vi "Dynamic Circle Find.vi"(8 "error in":errorcluster, 9 "Range":cluster{"Start":sgl, "Count":sgl}={"Start"=0.0, "Count"=255.0}, 10 "Treatment":T1, 11 "Images":T3) -> (0 "error out":errorcluster, 2 "Circle":T4, 3 "Found":bool)   [LabVIEW 2015]
uses:
  controls/Results.ctl
  controls/Images.ctl
  <vilib>/vision/Image Controls.llb/IMAQ Image.ctl
  controls/Treatment Parameters.ctl
  <vilib>/vision/NI_Vision_Development_Module.lvlib
panel:
  out "Array":sgl[][](array[numeric])
  out "Template":T2(plugin-control)
  out "Buffer":T2(plugin-control)
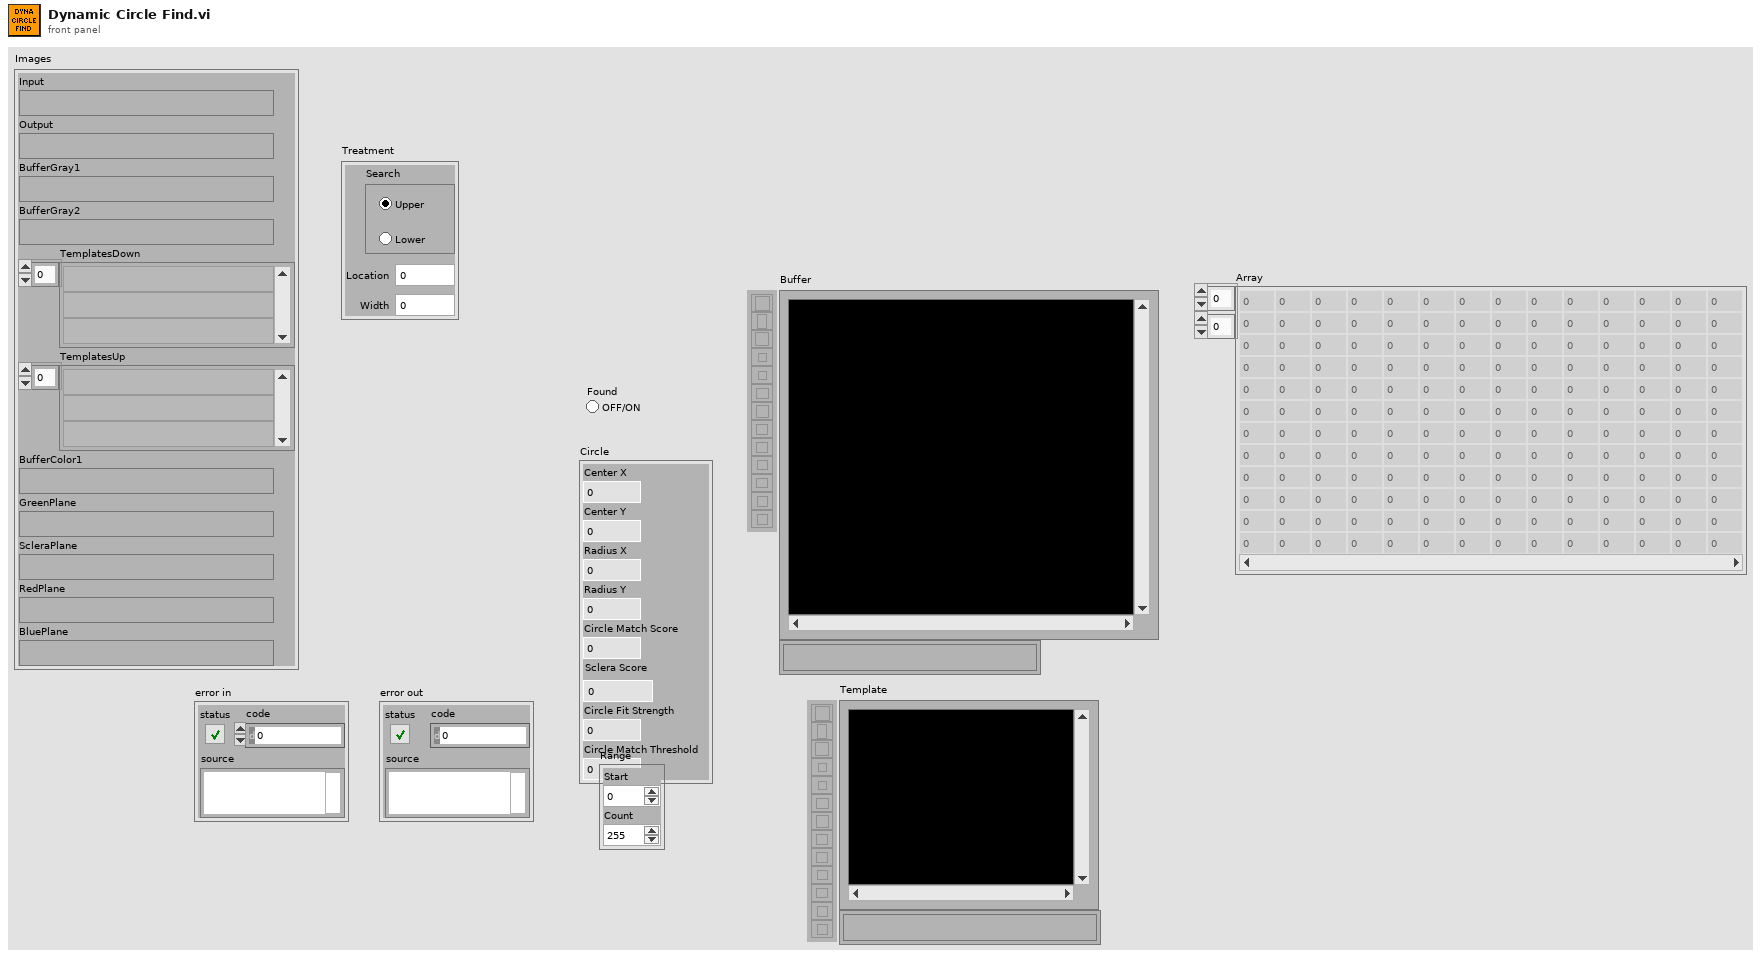
[diagram p1: front panel]
types:
  T1 = typedef "Treatment Parameters.ctl" = cluster{"Location":dbl, "Width":dbl, "Search":enum32{"Upper", "Lower"}}
  T2 = typedef "IMAQ Image.ctl" = refnum<image>
  T3 = typedef "Images.ctl" = cluster{"Input":T2, "Output":T2, "BufferGray1":T2, "BufferGray2":T2, "TemplatesDown":T2[], "TemplatesUp":T2[], "BufferColor1":T2, "GreenPlane":T2, "ScleraPlane":T2, "RedPlane":T2, "BluePlane":T2}
  T4 = typedef "Results.ctl" = cluster{"Center X":i32, "Center Y":i32, "Radius X":i32, "Radius Y":i32, "Circle Match Score":i32, "Sclera Score":dbl, "Circle Fit Strength":i32, "Circle Match Threshold":i32}
  T5 = cluster{"Global Rectangle":i32[], "Contours":cluster{"ID":enum32{"External", "Internal"}, "Type":u32, "Coordinates":i32[]}[]}
  T6 = cluster{"Number of Matches Requested":i32, "Minimum Match Score":sgl, "Angle Ranges":cluster{"Start Angle":sgl, "End Angle":sgl}[]}
  T7 = cluster{"histogram":u32[], "Minimal Value":sgl, "Maximal Value":sgl, "Starting Value":sgl, "Interval Width":sgl, "Mean Value":sgl, "Standard  Variation":sgl, "Area (pixels)":i32}
  T8 = typedef "Image Type" = u32
  T9 = cluster{"Position":cluster{"x":sgl, "y":sgl}, "Angle":sgl, "Scale":sgl, "Score":sgl, "Bounding Box":cluster{"x":sgl, "y":sgl}[]}[]
  T10 = cluster{"Position":cluster{"x":sgl, "y":sgl}, "Angle":sgl, "Scale":sgl, "Score":sgl, "Bounding Box":cluster{"x":sgl, "y":sgl}[]}
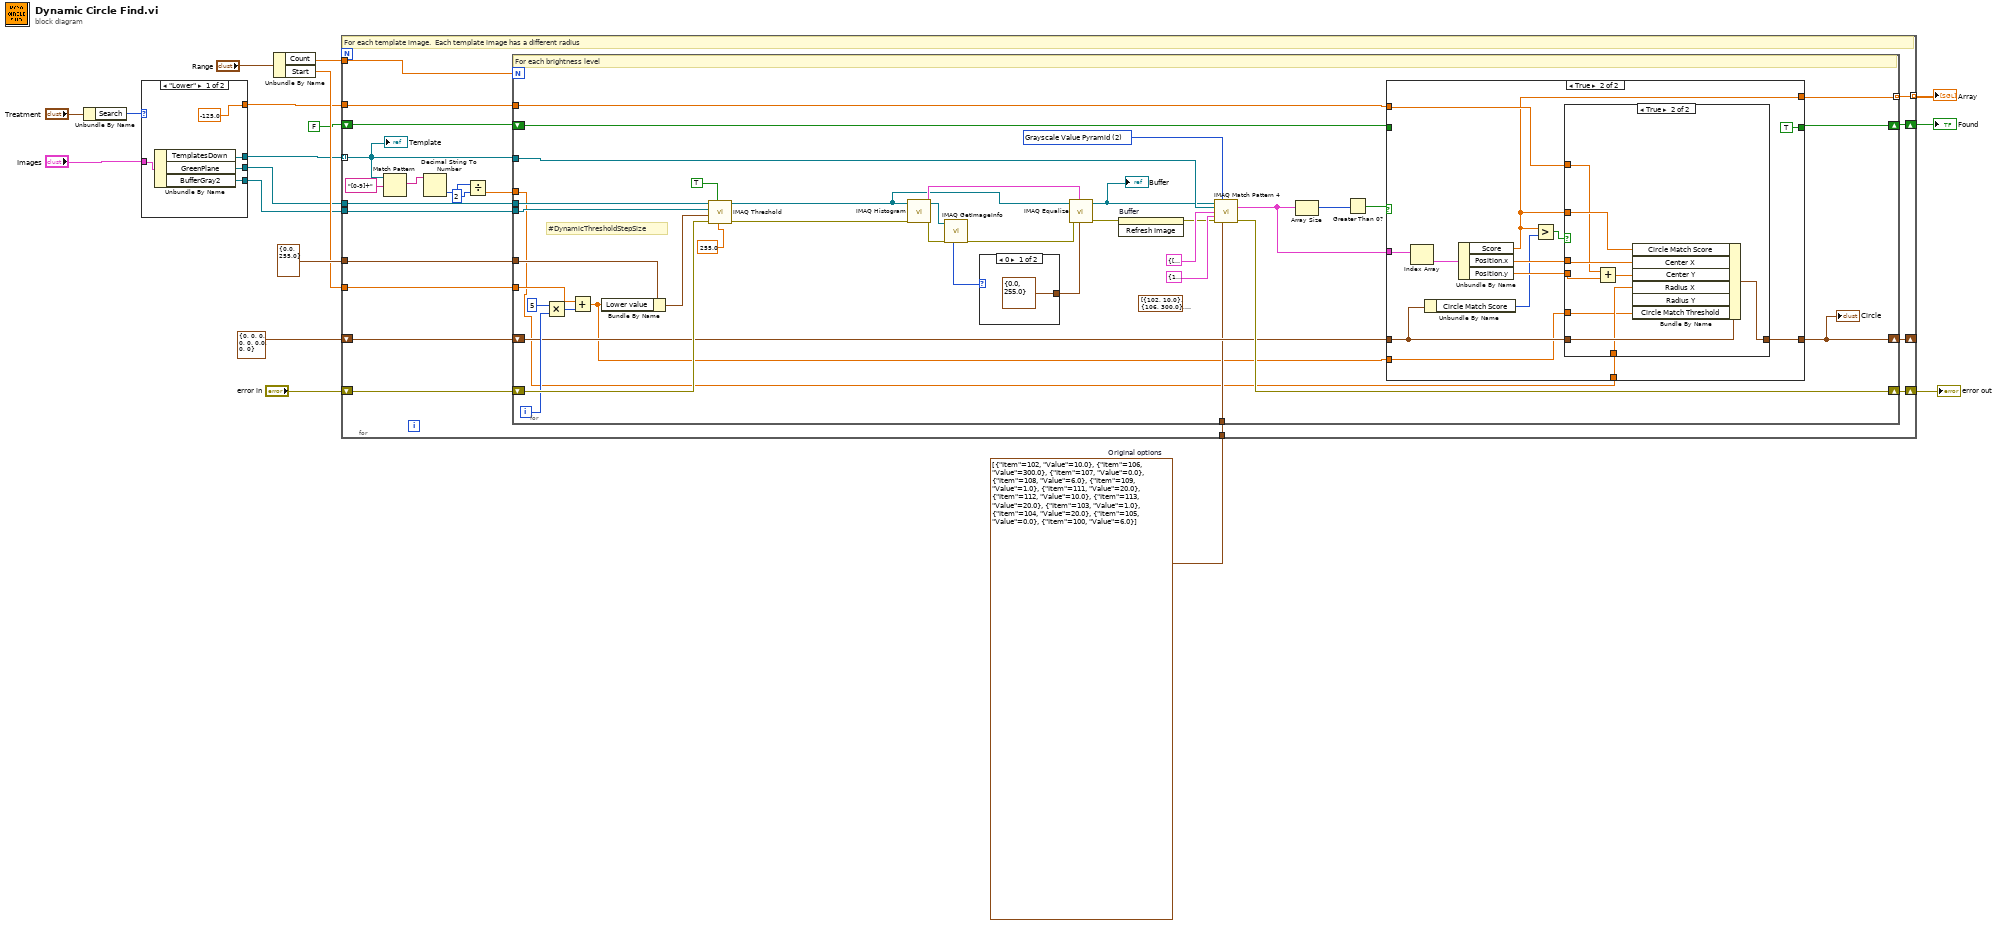
[diagram p0: block diagram]
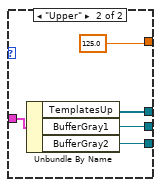
[diagram p2: hidden frame]
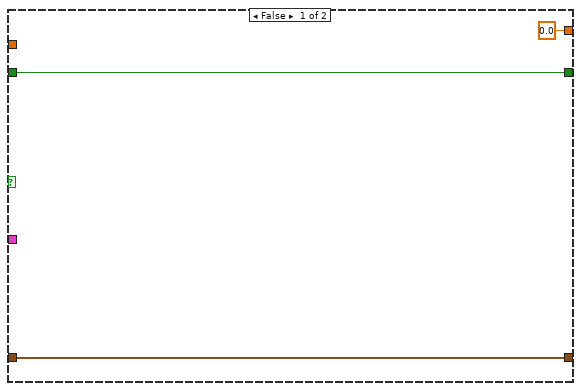
[diagram p3: hidden frame]
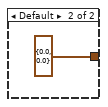
[diagram p5: hidden frame]
diagram:
  w3 = cluster{"Item":u16, "Value":dbl}[] [{"Item"=102, "Value"=10.0}, {"Item"=106, "Value"=300.0}, {"Item"=107, "Value"=0.0}, {"Item"=108, "Value"=6.0}, {"Item"=109, "Value"=1.0}, {"Item"=111, "Value"=20.0}, {"Item"=112, "Value"=10.0}, {"Item"=113, "Value"=20.0}, {"Item"=103, "Value"=1.0}, {"Item"=104, "Value"=20.0}, {"Item"=105, "Value"=0.0}, {"Item"=100, "Value"=6.0}]  # Original options
  n1 = Unbundle By Name("Treatment") -> ("Search"=w5:enum32{"Upper", "Lower"})
  n2 = case shown="\"Lower\"" w5 {
    tunnel: "Images" -> [w23 w28]
    tunnel: [w22 w27] -> w8
    tunnel: [w21 w26] -> w7
    tunnel: [w20 w25] -> w4
    tunnel: [sgl -125.0 ("Lower value") sgl 125.0 ("Lower value")] -> w2
    frame "Lower" {
      n3 = Unbundle By Name(w23) -> ("TemplatesDown"=w22:T2[], "GreenPlane"=w21:T2, "BufferGray2"=w20:T2)
    }
    frame "Upper" {
      n4 = Unbundle By Name(w28) -> ("TemplatesUp"=w27:T2[], "BufferGray1"=w26:T2, "BufferGray2"=w25:T2)
    }
  }
  n5 = Unbundle By Name("Range") -> ("Count"=w14:sgl, "Start"=w13:sgl)
  n6 = for {
    tunnel: cluster{"Lower value":sgl, "Upper value":sgl} {"Lower value"=0.0, "Upper value"=255.0} ("Range (Threshold 1)") -> [w47]
    tunnel: w7 -> [w46]
    tunnel: w14 -> [w45]
    tunnel: w13 -> [w44]
    tunnel: w8 -> [w34] mode=indexing
    shift-right: [w48] -> w18
    shift-left: "error in" -> [w40]
    shift-right: [w37] -> _
    shift-left: T4 {"Center X"=0, "Center Y"=0, "Radius X"=0, "Radius Y"=0, "Circle Match Score"=0, "Sclera Score"=0.0, "Circle Fit Strength"=0, "Circle Match Threshold"=0} -> [w43]
    shift-right: [w41] -> w10
    shift-left: FALSE -> [w42]
    tunnel: w4 -> [w39]
    tunnel: w3 -> [w38]
    tunnel: w2 -> [w36]
    tunnel: [w35] -> w1 mode=indexing
    # "For each template image.  Each template image has a different radius"
    n7 = Match Pattern(string=w34, regular expression="[0-9]+") -> (match substring=w29:string)  [unwired: 1 in, 3 out]
    n8 = Decimal String To Number(string=w29) -> (number=w32:i32)  [unwired: 2 in, 1 out]
    n9 = Divide(x=w32, y=2 ("x")) -> (x/y=w31:dbl)
    n10 = for {
      N: w45 -> [_]
      tunnel: w47 -> [w75]
      tunnel: w46 -> [w73]
      shift-right: [w84] -> w48
      shift-left: w40 -> [w72]
      tunnel: w44 -> [w68]
      shift-right: [w53] -> w37
      shift-left: w43 -> [w66]
      shift-right: [w63] -> w41
      shift-left: w42 -> [w64]
      tunnel: w34 -> [w62]
      tunnel: w39 -> [w60]
      tunnel: w38 -> [w54]
      tunnel: w36 -> [w52]
      tunnel: [w51] -> w35 mode=indexing
      tunnel: w31 -> [w50]
      i -> [w70]
      w83 = 2 items=["All", "Low Discrepancy Sampling", "Grayscale Value Pyramid", "Gradients Pyramid"] ("Algorithm")
      (unwired) cluster{"Item":u16, "Value":dbl}[] [{"Item"=102, "Value"=10.0}, {"Item"=106, "Value"=300.0}, {"Item"=107, "Value"=0.0}, {"Item"=108, "Value"=6.0}, {"Item"=109, "Value"=1.0}, {"Item"=111, "Value"=20.0}, {"Item"=112, "Value"=10.0}, {"Item"=113, "Value"=20.0}, {"Item"=103, "Value"=1.0}, {"Item"=104, "Value"=20.0}, {"Item"=105, "Value"=0.0}, {"Item"=100, "Value"=6.0}] ("Advanced Options")
      # "#DynamicThresholdStepSize"
      # "For each brightness level"
      n11 = Multiply(x=5, y=w70) -> (x*y=w69:i32)
      n12 = Add(x=w68, y=w69) -> (x+y=w49:sgl)
      n13 = Bundle By Name(cluster=w75, "Lower value"=w49) -> (w71:cluster{"Lower value":sgl, "Upper value":sgl})
      n14 = call "IMAQ Threshold"("Replace Value"=sgl 255.0, "Keep/Replace Value (Replace)"=TRUE, "error in (no error)"=w72, "Range"=w71, "Image Dst"=w60, "Image Src"=w73) -> ("error out"=w58:errorcluster, "Image Dst Out"=w74:T2)  [unwired: 4 out]
      n15 = call "IMAQ Histogram"("error in (no error)"=w58, "Image"=w74) -> ("error out"=w78:errorcluster, "Histogram Report"=w76:T7)  [unwired: 3 in, 5 out]
      n16 = call "IMAQ GetImageInfo"("error in (no error)"=w78, "Image"=w74) -> ("error out"=w79:errorcluster, "Image Type"=w77:T8)  [unwired: 8 out]
      n17 = case shown="0" w77 {
        tunnel: [cluster{"Minimum":sgl, "Maximum":sgl} {"Minimum"=0.0, "Maximum"=255.0} ("Range") cluster{"Minimum":sgl, "Maximum":sgl} {"Minimum"=0.0, "Maximum"=0.0} ("Range")] -> w80
        frame 0 {
        }
        frame Default {
        }
      }
      n18 = call "IMAQ Equalize"("Range"=w80, "Histogram Report"=w76, "error in (no error)"=w79, "Image Src"=w74) -> ("error out"=w57:errorcluster, "Image Dst Out"=w55:T2)  [unwired: 2 in, 4 out]
      "Buffer" <- w55
      n19 = invoke on="Buffer" class="ImageControl" method="Refresh Image"(error in=w57) -> (error out=w56:errorcluster)  [unwired: 2 in, 2 out]
      n20 = call "IMAQ Match Pattern 4"("Image"=w55, "Algorithm"=w83, "Template Image"=w62, "ROI Descriptor"=T5 {"Global Rectangle"=[0, 0, 1279, 1023], "Contours"=[{"ID"=enum."External", "Type"=12, "Coordinates"=[0, 0, 1279, 1023, 0]}]}, "Parameters"=T6 {"Number of Matches Requested"=1, "Minimum Match Score"=0.0, "Angle Ranges"=[]}, "error in (no error)"=w56, "Advanced Options"=w54) -> ("Matches (pixel)"=w85:T9, "error out"=w84:errorcluster)  [unwired: 4 in, 3 out]
      n21 = Array Size(array=w85) -> (size(s)=w86:i32)
      n22 = Greater Than 0?(x=w86) -> (x > 0?=w65:bool)
      n23 = case shown="True" w65 {
        tunnel: w85 -> [_ w102]
        tunnel: [w89 w101] -> w53
        tunnel: w66 -> [w89 w95]
        tunnel: w64 -> [w88 _]
        tunnel: [w88 TRUE] -> w63
        tunnel: w50 -> [_ w93]
        tunnel: w52 -> [_ w92]
        tunnel: [sgl 0.0 ("Score") w91] -> w51
        tunnel: w49 -> [_ w90]
        frame False {
        }
        frame True {
          n24 = Index Array(array=w102) -> (element=w98:T10)  [unwired: 1 in]
          n25 = Unbundle By Name(w95) -> ("Circle Match Score"=w94:i32)
          n26 = Unbundle By Name(w98) -> ("Score"=w91:sgl, "Position.x"=w99:sgl, "Position.y"=w100:sgl)
          n27 = Greater?(x=w91, y=w94) -> (0:w97:bool)
          n28 = case shown="True" w97 {
            tunnel: [w103 w112] -> w101
            tunnel: w100 -> [_ w111]
            tunnel: w99 -> [_ w110]
            tunnel: w95 -> [w103 w109]
            tunnel: w91 -> [_ w108]
            tunnel: w93 -> [_ w107]
            tunnel: w92 -> [_ w105]
            tunnel: w90 -> [_ w104]
            frame False {
            }
            frame True {
              n29 = Add(x=w105, y=w111) -> (x+y=w106:sgl)
              n30 = Bundle By Name(cluster=w109, "Circle Match Score"=w108, "Center X"=w110, "Center Y"=w106, "Radius X"=w107, "Radius Y"=w107, "Circle Match Threshold"=w104) -> (w112:T4)
            }
          }
        }
      }
      "Circle" <- w53
    }
    "Template" <- w34
  }
  "Found" <- w10
  "error out" <- w18
  "Array" <- w1
